vi "Main Tclk.vi"() -> ()   [LabVIEW 2018] (continued)
                n1472 = Multiply(x=w6714, y=w6704) -> (x*y=w6715:dbl)
                n1473 = local read "X full scale (V)"() -> (w6718:sgl)
                n1474 = Subtract(x=w6750, y="Y shift (nm/image)") -> (x-y=w6744:dbl)
                n1475 = expression code="x/1000"(w6744) -> (w6743:dbl)
                n1476 = Max & Min(x=0.1 ("upper limit"), y=w6715) -> (max(x,y)=w6708:dbl, min(x,y)=w6707:dbl)
                n1477 = Multiply(x=w6721, y=w6718) -> (x*y=w6722:dbl)
                n1478 = expression code="x/1000"("X shift (nm/image)") -> (w6745:sgl)
                n1479 = Select(t=w6722, s=w6720, f=w6717) -> (s? t:f=w6709:dbl)
                n1480 = Subtract(x=w6726, y=w6743) -> (x-y=w6753:dbl)
                n1481 = In Range and Coerce(upper limit=w6708, x=w6709, lower limit=w6707) -> (coerced(x)=w6705:dbl)  [unwired: 1 out]
                n1482 = Add(x=w6727, y=w6745) -> (x+y=w6748:sgl)
                n1483 = Multiply(x=w6703, y=w6704) -> (x*y=w6706:dbl)
                n1484 = Divide(x=w6706, y=w6705) -> (x/y=w6702:dbl)
                n1485 = Subtract(x=w6702, y=w6703) -> (x-y=w6742:dbl)
                n1486 = Subtract(x=w6702, y=w6710) -> (x-y=w6739:dbl)
                n1487 = expression code="x/2"(w6742) -> (w6741:dbl)
                n1488 = expression code="x/2"(w6739) -> (w6738:dbl)
                n1489 = Negate(x=w6741) -> (-x=w6740:dbl)
                n1490 = Negate(x=w6738) -> (-x=w6737:dbl)
                n1491 = In Range and Coerce(upper limit=w6741, x=w6748, lower limit=w6740) -> (coerced(x)=w6747:dbl)  [unwired: 1 out]
                n1492 = In Range and Coerce(upper limit=w6738, x=w6753, lower limit=w6737) -> (coerced(x)=w6752:dbl)  [unwired: 1 out]
                n1493 = local read "SEM Scan Parameters"() -> (w6757:T26)
                n1494 = Bundle By Name(cluster=w6757, "WD (mm)"=w6735, "X stig"=w6734, "Y stig"=w6733, "X aln"=w6732, "Y aln"=w6731, "X center (um)"=w6747, "Y center (um)"=w6752) -> (w6756:T26)
                n1495 = local write "SEM Scan Parameters"(w6756) -> ()
              }
              frame #17 {
                n1496 = local read "SEM Scan Parameters"() -> (w6879:T26)
                n1497 = local read "AF Count"() -> (w6875:u8)
                n1498 = local read "Auto Focus"() -> (w6881:bool)
                n1499 = Unbundle By Name(w6879) -> ("WD (mm)"=w6880:sgl[][])
                n1500 = case shown="True" w6881 {
                  tunnel: w6880 -> [w6889 w6899]
                  tunnel: [w6886 w6894] -> w6878
                  tunnel: [sgl[][][] [] ("Array") w6895] -> w6876
                  tunnel: w6875 -> [_ w6896]
                  frame False {
                    n1501 = local read "Milling para"() -> (w6891:T35)
                    n1502 = To Double Precision Float(number=w6889) -> (double precision float=w6885:dbl[][])
                    n1503 = Unbundle By Name(w6891) -> ("Z-step (nm)"=w6884:dbl, "Lines auto pause"=w6882:u16)
                    n1504 = expression code="1/sin(x/180*pi)"("FIB-SEM Angle") -> (w6890:dbl)
                    n1505 = expression code="x/1e6"(w6884) -> (w6883:dbl)
                    n1506 = Compound Arithmetic op=MULTIPLY(w6883, w6882, w6890) -> (w6893:dbl)
                    n1507 = Add(x=w6885, y=w6893) -> (x+y=w6888:dbl[][])
                    n1508 = To Single Precision Float(number=w6888) -> (single precision float=w6886:sgl[][])
                  }
                  frame True {
                    n1509 = property on="AF Steps" class="DigNum (strict)"("DisabledEnum"=T44."Disabled and Grayed Out" ("Disabled")) -> ()  [unwired: 2 in, 2 out]
                    n1510 = for {
                      tunnel: w6896 -> [w6905]
                      tunnel: w6899 -> [w6904] mode=indexing
                      tunnel: [w6903] -> w6898 mode=indexing
                      tunnel: [w6902] -> w6897 mode=indexing
                      i -> [w6901]
                      n1511 = for {
                        tunnel: w6905 -> [w6910]
                        tunnel: w6904 -> [w6913] mode=indexing
                        tunnel: [w6912] -> w6903 mode=indexing
                        tunnel: [w6911] -> w6902 mode=indexing
                        tunnel: w6901 -> [w6908]
                        i -> [w6906]
                        n1512 = Decrement(x=w6910) -> (x-1=w6907:u8)
                        n1513 = Equal To 0?(x=w6907) -> (x = 0?=w6909:bool)
                        n1514 = case shown="True" w6909 {
                          tunnel: [w6917 w6921] -> w6914
                          tunnel: w6913 -> [_ w6922]
                          tunnel: [w6917 w6921] -> w6911
                          tunnel: w6908 -> [w6916 _]
                          tunnel: w6906 -> [w6915 _]
                          frame False {
                            n1515 = local read "WD array tiled"() -> (w6918:sgl[][][])
                            n1516 = Index Array(array=w6918, index (dim 0)=w6916, index (dim 1)=w6915) -> (element=w6917:sgl[])  [unwired: 1 in]
                          }
                          frame True {
                            n1517 = local read "AF Range (nm)"() -> (w6920:sgl)
                            n1518 = local read "AF Steps"() -> (w6919:u8)
                            n1519 = expression code="x/1e6"(w6920) -> (w6923:sgl)
                            n1520 = call "Step down array.vi"("Steps"=w6919, "Range"=w6923, "Center"=w6922) -> ("Array"=w6921:dbl[])  [unwired: 8 in]
                          }
                        }
                        n1521 = Index Array(array=w6914, index=w6907) -> (element=w6912:dbl)
                      }
                    }
                    n1522 = To Single Precision Float(number=w6897) -> (single precision float=w6895:sgl[][][])
                    n1523 = To Single Precision Float(number=w6898) -> (single precision float=w6894:sgl[][])
                  }
                }
                n1524 = Bundle By Name(cluster=w6879, "WD (mm)"=w6878) -> (w6877:T26)
                n1525 = local write "WD array tiled"(w6876) -> ()
                n1526 = local write "SEM Scan Parameters"(w6877) -> ()
              }
              frame #18 {
                n1527 = local read "SEM Scan Parameters"() -> (w6931:T26)
                n1528 = local read "AS Count"() -> (w6925:u8)
                n1529 = local read "AA Count"() -> (w6924:u8)
                n1530 = Unbundle By Name(w6931) -> ("X stig"=w6934:sgl[][], "Y stig"=w6935:sgl[][])
                n1531 = Unbundle By Name(w6931) -> ("X aln"=w6937:sgl[][], "Y aln"=w6938:sgl[][])
                n1532 = case shown="\"Stig X\"" "Stig Options" {
                  tunnel: [w7005 w7012 w7038] -> w6930
                  tunnel: [w7004 w7009 w7040] -> w6929
                  tunnel: w6934 -> [w7005 w7010 w7038]
                  tunnel: w6935 -> [w7004 w7009 w7039]
                  tunnel: [w7003 w7008 dbl[][][] [] ("Array")] -> w6936
                  tunnel: [w7003 dbl[][][] [] ("Array") w7037] -> w6939
                  tunnel: w6925 -> [_ w7007 w7036]
                  frame "Defaut", Default {
                    w7003 = dbl[][][] [] ("Array")
                  }
                  frame "Stig X" {
                    n1533 = property on="AS Steps" class="DigNum (strict)"("DisabledEnum"=T44."Disabled and Grayed Out" ("Disabled")) -> ()  [unwired: 2 in, 2 out]
                    n1534 = for {
                      tunnel: w7007 -> [w7017]
                      tunnel: [w7016] -> w7012 mode=indexing
                      tunnel: w7010 -> [w7015] mode=indexing
                      tunnel: [w7014] -> w7008 mode=indexing
                      i -> [w7013]
                      n1535 = for {
                        tunnel: w7017 -> [w7022]
                        tunnel: [w7025] -> w7016 mode=indexing
                        tunnel: w7015 -> [w7024] mode=indexing
                        tunnel: [w7023] -> w7014 mode=indexing
                        tunnel: w7013 -> [w7019]
                        i -> [w7018]
                        n1536 = Decrement(x=w7022) -> (x-1=w7020:u8)
                        n1537 = Equal To 0?(x=w7020) -> (x = 0?=w7021:bool)
                        n1538 = case shown="False" w7021 {
                          tunnel: [w7027 w7033] -> w7026
                          tunnel: w7024 -> [_ w7034]
                          tunnel: [w7027 w7033] -> w7023
                          tunnel: w7019 -> [w7029 _]
                          tunnel: w7018 -> [w7028 _]
                          frame False {
                            n1539 = local read "StigX array tiled"() -> (w7030:sgl[][][])
                            n1540 = Index Array(array=w7030, index (dim 0)=w7029, index (dim 1)=w7028) -> (element=w7027:sgl[])  [unwired: 1 in]
                          }
                          frame True {
                            n1541 = local read "AS Range (%)"() -> (w7032:sgl)
                            n1542 = local read "AS Steps"() -> (w7031:u8)
                            n1543 = call "Step down array.vi"("Steps"=w7031, "Range"=w7032, "Center"=w7034) -> ("Array"=w7033:dbl[])  [unwired: 8 in]
                          }
                        }
                        n1544 = Index Array(array=w7026, index=w7020) -> (element=w7025:dbl)
                      }
                    }
                  }
                  frame "Stig Y" {
                    n1545 = property on="AS Steps" class="DigNum (strict)"("DisabledEnum"=T44."Disabled and Grayed Out" ("Disabled")) -> ()  [unwired: 2 in, 2 out]
                    n1546 = for {
                      tunnel: w7036 -> [w7046]
                      tunnel: [w7045] -> w7040 mode=indexing
                      tunnel: [w7044] -> w7037 mode=indexing
                      tunnel: w7039 -> [w7043] mode=indexing
                      i -> [w7042]
                      n1547 = for {
                        tunnel: w7046 -> [w7050]
                        tunnel: [w7054] -> w7045 mode=indexing
                        tunnel: [w7053] -> w7044 mode=indexing
                        tunnel: w7043 -> [w7052] mode=indexing
                        tunnel: w7042 -> [w7048]
                        i -> [w7047]
                        n1548 = Decrement(x=w7050) -> (x-1=w7049:u8)
                        n1549 = Equal To 0?(x=w7049) -> (x = 0?=w7051:bool)
                        n1550 = case shown="False" w7051 {
                          tunnel: [w7056 w7061] -> w7055
                          tunnel: [w7056 w7061] -> w7053
                          tunnel: w7052 -> [_ w7060]
                          tunnel: w7048 -> [w7058 _]
                          tunnel: w7047 -> [w7057 _]
                          frame False {
                            n1551 = local read "StigY array tiled"() -> (w7059:sgl[][][])
                            n1552 = Index Array(array=w7059, index (dim 0)=w7058, index (dim 1)=w7057) -> (element=w7056:sgl[])  [unwired: 1 in]
                          }
                          frame True {
                            n1553 = local read "AS Range (%)"() -> (w7062:sgl)
                            n1554 = local read "AS Steps"() -> (w7063:u8)
                            n1555 = call "Step down array.vi"("Steps"=w7063, "Range"=w7062, "Center"=w7060) -> ("Array"=w7061:dbl[])  [unwired: 8 in]
                          }
                        }
                        n1556 = Index Array(array=w7055, index=w7049) -> (element=w7054:dbl)
                      }
                    }
                  }
                }
                n1557 = case shown="\"Aln Y\"" "Aln Options" {
                  tunnel: [w6944 w6951 w6979] -> w6928
                  tunnel: [w6943 w6947 w6977] -> w6927
                  tunnel: w6937 -> [w6944 w6949 w6979]
                  tunnel: w6938 -> [w6943 w6947 w6978]
                  tunnel: [w6942 w6948 dbl[][][] [] ("Array")] -> w6940
                  tunnel: [w6942 dbl[][][] [] ("Array") w6976] -> w6941
                  tunnel: w6924 -> [_ w6946 w6975]
                  frame "Defaut", Default {
                    w6942 = dbl[][][] [] ("Array")
                  }
                  frame "Aln X" {
                    n1558 = property on="AA Steps" class="DigNum (strict)"("DisabledEnum"=T44."Disabled and Grayed Out" ("Disabled")) -> ()  [unwired: 2 in, 2 out]
                    n1559 = for {
                      tunnel: [w6956] -> w6951 mode=indexing
                      tunnel: w6949 -> [w6955] mode=indexing
                      tunnel: [w6954] -> w6948 mode=indexing
                      tunnel: w6946 -> [w6953]
                      i -> [w6952]
                      n1560 = for {
                        tunnel: [w6964] -> w6956 mode=indexing
                        tunnel: w6955 -> [w6963] mode=indexing
                        tunnel: [w6962] -> w6954 mode=indexing
                        tunnel: w6953 -> [w6961]
                        tunnel: w6952 -> [w6958]
                        i -> [w6957]
                        n1561 = Decrement(x=w6961) -> (x-1=w6959:u8)
                        n1562 = Equal To 0?(x=w6959) -> (x = 0?=w6960:bool)
                        n1563 = case shown="False" w6960 {
                          tunnel: [w6966 w6972] -> w6965
                          tunnel: w6963 -> [_ w6973]
                          tunnel: [w6966 w6972] -> w6962
                          tunnel: w6958 -> [w6967 _]
                          tunnel: w6957 -> [w6968 _]
                          frame False {
                            n1564 = local read "AlnX array tiled"() -> (w6969:sgl[][][])
                            n1565 = Index Array(array=w6969, index (dim 0)=w6967, index (dim 1)=w6968) -> (element=w6966:sgl[])  [unwired: 1 in]
                          }
                          frame True {
                            n1566 = local read "AA Range (%)"() -> (w6970:sgl)
                            n1567 = local read "AA Steps"() -> (w6971:u8)
                            n1568 = call "Step down array.vi"("Steps"=w6971, "Range"=w6970, "Center"=w6973) -> ("Array"=w6972:dbl[])  [unwired: 8 in]
                          }
                        }
                        n1569 = Index Array(array=w6965, index=w6959) -> (element=w6964:dbl)
                      }
                    }
                  }
                  frame "Aln Y" {
                    n1570 = property on="AA Steps" class="DigNum (strict)"("DisabledEnum"=T44."Disabled and Grayed Out" ("Disabled")) -> ()  [unwired: 2 in, 2 out]
                    n1571 = for {
                      tunnel: w6975 -> [w6985]
                      tunnel: w6978 -> [w6984] mode=indexing
                      tunnel: [w6983] -> w6977 mode=indexing
                      tunnel: [w6982] -> w6976 mode=indexing
                      i -> [w6981]
                      n1572 = for {
                        tunnel: w6985 -> [w6990]
                        tunnel: w6984 -> [w6993] mode=indexing
                        tunnel: [w6992] -> w6983 mode=indexing
                        tunnel: [w6991] -> w6982 mode=indexing
                        tunnel: w6981 -> [w6987]
                        i -> [w6986]
                        n1573 = Decrement(x=w6990) -> (x-1=w6989:u8)
                        n1574 = Equal To 0?(x=w6989) -> (x = 0?=w6988:bool)
                        n1575 = case shown="False" w6988 {
                          tunnel: [w6995 w6999] -> w6994
                          tunnel: w6993 -> [_ w7000]
                          tunnel: [w6995 w6999] -> w6991
                          tunnel: w6987 -> [w6996 _]
                          tunnel: w6986 -> [w6997 _]
                          frame False {
                            n1576 = local read "AlnY array tiled"() -> (w6998:sgl[][][])
                            n1577 = Index Array(array=w6998, index (dim 0)=w6996, index (dim 1)=w6997) -> (element=w6995:sgl[])  [unwired: 1 in]
                          }
                          frame True {
                            n1578 = local read "AA Steps"() -> (w7002:u8)
                            n1579 = local read "AA Range (%)"() -> (w7001:sgl)
                            n1580 = call "Step down array.vi"("Steps"=w7002, "Range"=w7001, "Center"=w7000) -> ("Array"=w6999:dbl[])  [unwired: 8 in]
                          }
                        }
                        n1581 = Index Array(array=w6994, index=w6989) -> (element=w6992:dbl)
                      }
                    }
                  }
                }
                n1582 = local write "StigX array tiled"(w6936) -> ()
                n1583 = local write "StigY array tiled"(w6939) -> ()
                n1584 = local write "AlnX array tiled"(w6940) -> ()
                n1585 = local write "AlnY array tiled"(w6941) -> ()
                n1586 = Bundle By Name(cluster=w6931, "X stig"=w6930, "Y stig"=w6929, "X aln"=w6928, "Y aln"=w6927) -> (w6926:T26)
                n1587 = local write "SEM Scan Parameters"(w6926) -> ()
              }
              frame #19 {
                n1588 = local read "Tiled scan inputs"() -> (w7073:T6)
                n1589 = local read "SEM HW Config"() -> (w7074:T9)
                n1590 = local read "Detector Information"() -> (w7075:T8)
                n1591 = local read "SEM Scan Parameters"() -> (w7076:T26)
                n1592 = local read "SEM Options"() -> (w7077:T27)
                n1593 = local read "Focus Index Options"() -> (w7071:T28)
                n1594 = local read "File Information"() -> (w7078:T31)
                n1595 = local read "SEM-FIB Delay (s)"() -> (w7066:u32)
                n1596 = local read "After SEM"() -> (w7069:bool)
                n1597 = local read "FIB"() -> (w7068:bool)
                n1598 = local read "Milling para"() -> (w7079:T35)
                n1599 = local read "Additional Info"() -> (w7064:cluster{"Restart flag":u8, "Stage move flag":u8})
                n1600 = Not(x=w7069) -> (.not. x?=w7065:bool)
                n1601 = Greater Than 0?(x=w7066) -> (x > 0?=w7067:bool)
                n1602 = Compound Arithmetic op=AND(w7067, w7065, w7068) -> (w7070:bool)
                n1603 = Bundle By Name(cluster=w7073, "HW Config"=w7074, "Det Info"=w7075, "SEM Scan Parameters"=w7076, "SEM Options"=w7077, "Focus Index Options"=w7071, "File Information"=w7078, "Milling para"=w7079, "Additional Info"=w7064) -> (w7072:T6)
                n1604 = case shown="True" w7070 {
                  tunnel: w7066 -> [_ w7080]
                  frame False {
                  }
                  frame True {
                    n1605 = local read "FIB blank condenser %"() -> (w7089:u8)
                    n1606 = expression code="x*10"(w7080) -> (w7081:u32)
                    n1607 = Number To Decimal String(number=w7080) -> (decimal integer string=w7082:string)  [unwired: 1 in]
                    n1608 = for {
                      N: w7081 -> [_]
                      stop <- w7092 stop-if-true
                      n1609 = local read "Mill Manual Pause"() -> (w7093:bool)
                      n1610 = local read "FIB"() -> (w7095:bool)
                      n1611 = Wait Until Next ms Multiple(millisecond multiple=u32 100) -> ()  [unwired: 1 out]
                      n1612 = Not(x=w7095) -> (.not. x?=w7094:bool)
                      n1613 = Or(x=w7094, y=w7093) -> (x .or. y?=w7092:bool)
                    }
                    n1614 = Less?(x=w7089, y=u8 100) -> (x < y?=w7091:bool)
                    n1615 = Greater Or Equal?(x=w7080, y=5.0) -> (x >= y?=w7090:bool)
                    n1616 = To Single Precision Float(number=w7089) -> (single precision float=w7088:sgl)
                    n1617 = Compound Arithmetic op=AND(w7091, w7090) -> (w7087:bool)
                    n1618 = Concatenate Strings(w7082, " s delay after FIB milling..." ("string")) -> (w7084:string)
                    n1619 = local write "Status message"(w7084) -> ()
                    n1620 = case shown="True" w7087 {
                      tunnel: w7088 -> [_ w7098]
                      tunnel: w7080 -> [_ w7097]
                      frame False {
                      }
                      frame True {
                        n1621 = stacked-sequence {
                          seq-local: [w7100 _ _ _] -> [_ w7108 _ _]
                          seq-local: [w7099 _ _ _] -> [_ w7106 _ w7117]
                          seq-local: [_ w7107 _ _] -> [_ _ _ w7118]
                          tunnel: w7098 -> [_ w7105 _ _]
                          tunnel: w7097 -> [_ _ w7111 _]
                          frame #0 {
                            n1622 = local read "Api"() -> (w7102:refnum<k7>)
                            n1623 = call "SmartSEM Remote API get float.vi"("lpszParam"="AP_FIB_CONDENSER" ("Status message"), "ActiveX Container"=w7102) -> ("vValue"=w7099:sgl, "reference out"=w7100:refnum<k7>)  [unwired: 7 in, 1 out]
                          }
                          frame #1 {
                            n1624 = Compound Arithmetic op=MULTIPLY(w7106, w7105, sgl 0.01 ("value")) -> (w7104:sgl)
                            n1625 = call "SmartSEM Remote API set float.vi"("vValue"=w7104, "lpszParam"="AP_FIB_CONDENSER" ("Status message"), "ActiveX Container"=w7108) -> ("reference out"=w7107:refnum<k7>)  [unwired: 7 in, 1 out]
                          }
                          frame #2 {
                            n1626 = expression code="(x-3)*10"(w7111) -> (w7110:u32)
                            n1627 = for {
                              N: w7110 -> [_]
                              stop <- w7112 stop-if-true
                              n1628 = local read "Mill Manual Pause"() -> (w7113:bool)
                              n1629 = local read "FIB"() -> (w7115:bool)
                              n1630 = Wait Until Next ms Multiple(millisecond multiple=u32 100) -> ()  [unwired: 1 out]
                              n1631 = Not(x=w7115) -> (.not. x?=w7114:bool)
                              n1632 = Or(x=w7114, y=w7113) -> (x .or. y?=w7112:bool)
                            }
                          }
                          frame #3 {
                            n1633 = call "SmartSEM Remote API set float.vi"("vValue"=w7117, "lpszParam"="AP_FIB_CONDENSER" ("Status message"), "ActiveX Container"=w7118) -> ()  [unwired: 7 in, 2 out]
                          }
                        }
                      }
                    }
                  }
                }
                n1634 = local write "Tiled scan inputs"(w7072) -> ()
              }
              frame #20 {
                n1635 = local read "Mill Stop"() -> (w7121:bool)
                n1636 = local read "FIB"() -> (w7124:bool)
                n1637 = local read "Stop"() -> (w7125:bool)
                n1638 = Not(x=w7125) -> (.not. x?=w7123:bool)
                n1639 = Not(x=w7121) -> (.not. x?=w7120:bool)
                n1640 = Compound Arithmetic op=AND(w7120, w7124, w7123) -> (w7122:bool)
                n1641 = case shown="True" w7122 {
                  frame False {
                  }
                  frame True {
                    w7182 = TRUE ("SEM Options.Set WD")
                    n1642 = local read "WatchDog Mode"() -> (w7144:u16)
                    n1643 = local read "Api"() -> (w7138:refnum<k7>)
                    n1644 = local read "Tiled scan inputs"() -> (w7186:T6)
                    n1645 = Bundle By Name(cluster=w7186, "SEM Options.Set WD"=w7182, "SEM Options.Set stig"=w7182, "SEM Options.Set aln"=w7182, "SEM Options.Freeze"=w7182) -> (w7139:T6)
                    n1646 = call "2D scan tiled.vi"("WatchDog Mode"=w7144, "Tiled scan inputs"=w7139, "ActiveX Container"=w7138) -> ("Image Focus Index Tiled"=w7181:T53, "Image Focus Index Array Tiled"=w7180:T54, "Low res scale Tiled (um/pix)"=→"Low res scale tiled":dbl[][], "Single scan outputs"=w7185:T55, "SEM Spec. I Tiled (nA)"=w7160:sgl[][], "8-bit over scale"=w7170:bool[])  [unwired: 3 in]
                    n1647 = Array Size(array=w7160) -> (size(s)=w7161:i32[])
                    n1648 = Multiply Array Elements(1:w7161) -> (0:w7162:i32)
                    n1649 = local read "FI Detector"() -> (w7194:u16)
                    n1650 = Reshape Array(w7160, w7162) -> (w7163:sgl[])
                    n1651 = call-poly <vilib>:"Mean.vi"("X"=w7163) -> ("mean"=→"SEM Specimen I":dbl)  [unwired: 1 out]
                    n1652 = Unbundle By Name(w7185) -> ("SEM Parameters"=w7184:T13, "Image Focus Index"=w7176:T14, "FIB parameters"=→"FIB Parameters":T56)
                    n1653 = case shown="0, Default" w7194 {
                      tunnel: w7181 -> [w7255 w7259 w7263 w7267]
                      tunnel: [w7254 w7256 w7262 w7266] -> w7204
                      tunnel: w7180 -> [w7253 w7258 w7261 w7265]
                      tunnel: [w7252 w7257 w7260 w7264] -> w7203
                      frame 0, Default {
                        n1654 = Unbundle By Name(w7255) -> ("A Img Focus Index"=w7254:sgl[][])
                        n1655 = Unbundle By Name(w7253) -> ("A Img Focus Index array"=w7252:sgl[][][][])
                      }
                      frame 1 {
                        n1656 = Unbundle By Name(w7259) -> ("B Img Focus Index"=w7256:sgl[][])
                        n1657 = Unbundle By Name(w7258) -> ("B Img Focus Index array"=w7257:sgl[][][][])
                      }
                      frame 2 {
                        n1658 = Unbundle By Name(w7263) -> ("C Img Focus Index"=w7262:sgl[][])
                        n1659 = Unbundle By Name(w7261) -> ("C Img Focus Index array"=w7260:sgl[][][][])
                      }
                      frame 3 {
                        n1660 = Unbundle By Name(w7267) -> ("D Img Focus Index"=w7266:sgl[][])
                        n1661 = Unbundle By Name(w7265) -> ("D Img Focus Index array"=w7264:sgl[][][][])
                      }
                    }
                    "Focus Index tiled" <- w7204
                    "Focus Index array tiled" <- w7203
                    n1662 = local read "Pause for reheat"() -> (w7137:bool)
                    n1663 = local write "SEM Parameters"(w7184) -> ()
                    n1664 = local write "Image Focus Index"(w7176) -> ()
                    n1665 = Index Array(array=w7170, index #1=0 ("index"), index #2=1 ("index")) -> (element #1=w7173:bool, element #2=w7174:bool)
                    n1666 = Select(t="Pausing for FIB reheat ..." ("Status message"), s=w7137, f="SEM between FIB" ("Status message")) -> (s? t:f=w7146:string)
                    n1667 = local write "Det A over scale"(w7173) -> ()
                    n1668 = local write "Det B over scale"(w7174) -> ()
                    n1669 = Array Size(array=w7204) -> (size(s)=w7179:i32[])
                    n1670 = Not(x=w7137) -> (.not. x?=w7133:bool)
                    n1671 = local write "Status message"(w7146) -> ()
                    n1672 = local read "SEM scan time"() -> (w7131:dbl)
                    n1673 = Multiply Array Elements(1:w7179) -> (0:w7178:i32)
                    n1674 = Reshape Array(w7204, w7178) -> (w7177:sgl[])
                    n1675 = call-poly <vilib>:"Mean.vi"("X"=w7177) -> ("mean"=→"Focus Index":dbl)  [unwired: 1 out]
                    n1676 = Greater Or Equal?(x=w7131, y=6.0) -> (x >= y?=w7135:bool)
                    n1677 = Less?(x="FIB blank condenser %", y=u8 100) -> (x < y?=w7130:bool)
                    n1678 = To Single Precision Float(number="FIB blank condenser %") -> (single precision float=w7127:sgl)
                    n1679 = Compound Arithmetic op=AND(w7130, w7133, w7135) -> (w7134:bool)
                    n1680 = case shown="True" w7134 {
                      tunnel: w7131 -> [w7205 w7220]
                      tunnel: [w7206 w7219] -> w7132
                      tunnel: w7127 -> [_ w7218]
                      frame False {
                        w7210 = 10.0 ("rate")
                        n1681 = In Range and Coerce(upper limit=60.0, x=w7205, lower limit=2.0) -> (coerced(x)=w7211:dbl)  [unwired: 1 out]
                        n1682 = Multiply(x=w7211, y=w7210) -> (x*y=w7212:dbl)
                        n1683 = for {
                          N: w7212 -> [_]
                          shift-right: [w7217] -> w7206
                          shift-left: sgl[][] [] -> [w7216]
                          tunnel: w7210 -> [w7214]
                          n1684 = shared-variable ".\\Zeiss Library.lvlib\\Logs"() -> (w7213:sgl[])  [unwired: 1 in, 1 out]
                          n1685 = expression code="1000/x"(w7214) -> (w7215:dbl)
                          n1686 = Wait Until Next ms Multiple(millisecond multiple=w7215) -> ()  [unwired: 1 out]
                          n1687 = Build Array (concatenate)(w7216, w7213) -> (w7217:sgl[][])
                        }
                      }
                      frame True {
                        n1688 = stacked-sequence {
                          seq-local: [w7222 _ _ _ _ _] -> [_ w7230 _ _ _ _]
                          seq-local: [w7221 _ _ _ _ _] -> [_ w7228 _ w7234 _ _]
                          seq-local: [_ w7229 _ _ _ _] -> [_ _ _ w7235 _ _]
                          tunnel: w7220 -> [_ _ w7233 _ _ _]
                          tunnel: [_ _ _ _ _ w7239] -> w7219
                          tunnel: w7218 -> [_ w7227 _ _ _ _]
                          frame #0 {
                            n1689 = local read "Api"() -> (w7224:refnum<k7>)
                            n1690 = call "SmartSEM Remote API get float.vi"("lpszParam"="AP_FIB_CONDENSER" ("Status message"), "ActiveX Container"=w7224) -> ("vValue"=w7221:sgl, "reference out"=w7222:refnum<k7>)  [unwired: 7 in, 1 out]
                          }
                          frame #1 {
                            n1691 = Compound Arithmetic op=MULTIPLY(w7228, w7227, sgl 0.01 ("value")) -> (w7226:sgl)
                            n1692 = call "SmartSEM Remote API set float.vi"("vValue"=w7226, "lpszParam"="AP_FIB_CONDENSER" ("Status message"), "ActiveX Container"=w7230) -> ("reference out"=w7229:refnum<k7>)  [unwired: 7 in, 1 out]
                          }
                          frame #2 {
                            n1693 = expression code="(x-4)*1000"(w7233) -> (w7232:dbl)
                            n1694 = Wait (ms)(milliseconds to wait=w7232) -> ()  [unwired: 1 out]
                          }
                          frame #3 {
                            n1695 = call "SmartSEM Remote API set float.vi"("vValue"=w7234, "lpszParam"="AP_FIB_CONDENSER" ("Status message"), "ActiveX Container"=w7235) -> ()  [unwired: 7 in, 2 out]
                          }
                          frame #4 {
                            n1696 = Wait (ms)(milliseconds to wait=u32 1000) -> ()  [unwired: 1 out]
                          }
                          frame #5 {
                            n1697 = for {
                              N: 20 -> [_]
                              shift-right: [w7244] -> w7239
                              shift-left: sgl[][] [] -> [w7243]
                              n1698 = shared-variable ".\\Zeiss Library.lvlib\\Logs"() -> (w7242:sgl[])  [unwired: 1 in, 1 out]
                              n1699 = Wait Until Next ms Multiple(millisecond multiple=u32 100) -> ()  [unwired: 1 out]
                              n1700 = Build Array (concatenate)(w7243, w7242) -> (w7244:sgl[][])
                            }
                          }
                        }
                      }
                    }
                    n1701 = shared-variable ".\\Zeiss Library.lvlib\\Faraday cup offset"() -> (w7165:sgl)  [unwired: 1 in, 1 out]
                    n1702 = local read "Alert Settings"() -> (w7158:T36)
                    n1703 = Unbundle By Name(w7158) -> ("Low limit (F)"=w7152:sgl, "High limit (F)"=w7153:sgl)
                    n1704 = local read "Machine Type"() -> (w7191:u8)
                    n1705 = local read "Faraday Cup array"() -> (w7202:sgl[])
                    n1706 = local read "Specimen I array"() -> (w7201:sgl[])
                    n1707 = shared-variable ".\\Zeiss Library.lvlib\\Specimen (nA)"() -> (w7143:sgl)  [unwired: 1 in, 1 out]
                    "Specimen I (nA)" <- w7143
                    n1708 = shared-variable ".\\Zeiss Library.lvlib\\Beam Dump 1 (nA)"() -> (w7142:sgl)  [unwired: 1 in, 1 out]
                    "Beam Dump 1 (nA)" <- w7142
                    n1709 = shared-variable ".\\Zeiss Library.lvlib\\Beam Dump 2 (nA)"() -> (w7141:sgl)  [unwired: 1 in, 1 out]
                    "Beam Dump 2 (nA)" <- w7141
                    n1710 = local read "Milling I array"() -> (w7167:sgl[])
                    n1711 = shared-variable ".\\Zeiss Library.lvlib\\Milling I (nA)"() -> (w7140:sgl)  [unwired: 1 in, 1 out]
                    "Milling I (nA)" <- w7140
                    n1712 = local read "Temp low limit array"() -> (w7156:sgl[])
                    n1713 = local read "Temp high limit array"() -> (w7155:sgl[])
                    n1714 = local read "Beam Dump 1 array"() -> (w7200:sgl[])
                    n1715 = local read "Beam Dump 2 array"() -> (w7168:sgl[])
                    n1716 = local read "Temp array"() -> (w7199:sgl[])
                    n1717 = local read "Temp (F)"() -> (w7187:sgl)
                    n1718 = shared-variable ".\\Zeiss Library.lvlib\\Temp (F)"(w7187) -> ()  [unwired: 1 in, 1 out]
                    n1719 = Build Array (concatenate)(w7201, w7143) -> (w7197:sgl[])
                    n1720 = Build Array (concatenate)(w7199, w7187) -> (w7192:sgl[])
                    n1721 = Build Array (concatenate)(w7200, w7142) -> (w7196:sgl[])
                    n1722 = Build Array (concatenate)(w7168, w7141) -> (w7169:sgl[])
                    n1723 = Build Array (concatenate)(w7167, w7140) -> (w7166:sgl[])
                    n1724 = Build Array (concatenate)(w7156, w7152) -> (w7157:sgl[])
                    n1725 = Build Array (concatenate)(w7155, w7153) -> (w7154:sgl[])
                    n1726 = Delete From Array(array=w7132, length=15.0 ("rate"), index (row)=0 ("disabled index (col)")) -> (array with subset deleted=w7151:sgl[][])  [unwired: 1 in, 1 out]
                    n1727 = local write "Temp array"(w7192) -> ()
                    n1728 = local write "Specimen I array"(w7197) -> ()
                    n1729 = local write "Milling I array"(w7166) -> ()
                    n1730 = local write "Temp low limit array"(w7157) -> ()
                    n1731 = local write "Temp high limit array"(w7154) -> ()
                    n1732 = local write "Beam Dump 1 array"(w7196) -> ()
                    n1733 = local write "Beam Dump 2 array"(w7169) -> ()
                    n1734 = Transpose 2D Array(2D array=w7151) -> (transposed array=w7193:sgl[][])
                    n1735 = for {
                      tunnel: [w7251] -> w7189 mode=indexing
                      tunnel: w7193 -> [w7250] mode=indexing
                      n1736 = call-poly <vilib>:"Basic Averaged DC-RMS.vi"("signal in"=w7250) -> ("DC value"=w7251:dbl)  [unwired: 7 in, 3 out]
                    }
                    n1737 = To Single Precision Float(number=w7189) -> (single precision float=w7195:sgl[])
                    n1738 = Index Array(array=w7195) -> (element=w7149:sgl)  [unwired: 1 in]
                    n1739 = Subtract(x=w7149, y=w7165) -> (x-y=w7190:sgl)
                    n1740 = case shown="2" w7191 {
                      tunnel: w7190 -> [w7245 _ _]
                      tunnel: [w7245 w7248 w7249] -> w7188
                      tunnel: w7142 -> [_ w7247 _]
                      tunnel: w7143 -> [_ w7246 _]
                      tunnel: w7149 -> [_ _ w7249]
                      frame 0, Default {
                      }
                      frame 1 {
                        n1741 = Subtract(x=w7247, y=w7246) -> (x-y=w7248:sgl)
                      }
                      frame 2 {
                      }
                    }
                    "Faraday Cup (nA)" <- w7188
                    n1742 = shared-variable ".\\Zeiss Library.lvlib\\Faraday Cup (nA)"(w7188) -> ()  [unwired: 1 in, 1 out]
                    n1743 = Build Array (concatenate)(w7202, w7188) -> (w7198:sgl[])
                    n1744 = local write "Faraday Cup array"(w7198) -> ()
                    "FRC resolution" <- sgl 0.0 ("FRC resolution")
                  }
                }
              }
              frame #21 {
                n1745 = local read "FI array for stop limit"() -> (w7309:sgl[])
                n1746 = local read "Focus Index"() -> (w7279:sgl)
                n1747 = local read "Milling para"() -> (w7276:T35)
                n1748 = local read "Machine Type"() -> (w7275:u8)
                n1749 = local read "Alert Settings"() -> (w7300:T36)
                n1750 = Unbundle By Name(w7276) -> ("FIB PID measured"=w7277:u8, "FIB PID target"=w7268:sgl)
                n1751 = Unbundle By Name(w7300) -> ("FI stop limit auto"=w7303:bool)
                n1752 = local read "Auto re-engage"() -> (w7272:bool)
                n1753 = Build Array (concatenate)(w7309, w7279) -> (w7301:sgl[])
                n1754 = Unbundle By Name(w7300) -> ("FI low limit auto"=w7307:bool)
                n1755 = local write "FI array for stop limit"(w7301) -> ()
                n1756 = Array Size(array=w7301) -> (size(s)=w7306:i32)
                n1757 = case shown="2" w7277 {
                  tunnel: w7275 -> [w7342 _ w7346 _]
                  tunnel: [w7341 0.5 ("Minimum half range") w7347 0.5 ("Minimum half range")] -> w7274
                  frame 0 {
                    n1758 = case shown="2" w7342 {
                      tunnel: [0.5 ("Minimum half range") 0.8 ("Minimum half range")] -> w7341
                      frame 0, Default {
                      }
                      frame 2 {
                      }
                    }
                  }
                  frame 1 {
                  }
                  frame 2 {
                    n1759 = case shown="2" w7346 {
                      tunnel: [0.3 ("Minimum half range") 0.6 ("Minimum half range")] -> w7347
                      frame 0, Default {
                      }
                      frame 2 {
                      }
                    }
                  }
                  frame 3, Default {
                  }
                }
                n1760 = Or(x=w7303, y=w7272) -> (x .or. y?=w7302:bool)
                n1761 = Greater Or Equal?(x=w7306, y=5 ("x")) -> (x >= y?=w7304:bool)
                n1762 = And(x=w7304, y=w7302) -> (x .and. y?=w7271:bool)
                n1763 = And(x=w7304, y=w7307) -> (x .and. y?=w7308:bool)
                n1764 = local read "Focus index array"() -> (w7286:sgl[])
                n1765 = case shown="True" w7308 {
                  tunnel: w7300 -> [w7351 w7361]
                  tunnel: w7301 -> [_ w7358]
                  tunnel: [w7351 w7352] -> w7270
                  frame False {
                  }
                  frame True {
                    w7357 = 0.2 ("Minimum half range")
                    n1766 = call "Auto limits.vi"("lower band factor"=w7357, "upper band factor"=w7357, "Method"="sqrt of mean", "Minimum half range"=0.1, "Length"=5, "Input array"=w7358) -> ("Low limit"=w7356:dbl)  [unwired: 3 in, 2 out]
                    n1767 = Max & Min(x=w7356, y=0.0) -> (max(x,y)=w7353:dbl)  [unwired: 1 out]
                    n1768 = Bundle By Name(cluster=w7361, "Focus index low limit"=w7353) -> (w7352:T36)
                    n1769 = local write "Alert Settings"(w7352) -> ()
                  }
                }
                n1770 = case shown="True" w7271 {
                  tunnel: w7270 -> [_ w7312]
                  tunnel: w7301 -> [_ w7319]
                  frame False {
                  }
                  frame True {
                    w7314 = 0.4 ("Minimum half range")
                    n1771 = call "Auto limits.vi"("lower band factor"=w7314, "upper band factor"=w7314, "Method"="sqrt of mean", "Minimum half range"=0.4, "Length"=10, "Input array"=w7319) -> ("Low limit"=w7318:dbl)  [unwired: 3 in, 2 out]
                    n1772 = Unbundle By Name(w7312) -> ("Focus index low limit"=w7311:sgl)
                    n1773 = Max & Min(x=w7318, y=0.0) -> ()  [unwired: 2 out]
                    n1774 = expression code="x*0.75"(w7311) -> (w7310:sgl)
                    n1775 = Bundle By Name(cluster=w7312, "Focus index stop limit"=w7310) -> (w7320:T36)
                    n1776 = local write "Alert Settings"(w7320) -> ()
                  }
                }
                n1777 = case shown="True" w7272 {
                  tunnel: [w7322 w7328] -> w7273
                  tunnel: w7274 -> [w7322 w7329]
                  tunnel: [1.0 ("Minimum half range") w7327] -> w7269
                  tunnel: w7268 -> [_ w7326]
                  frame False {
                  }
                  frame True {
                    n1778 = local read "Re-engage counts"() -> (w7330:u8)
                    n1779 = expression code="x*0.15"(w7326) -> (w7325:sgl)
                    n1780 = Max & Min(x=sgl 1.0, y=w7325) -> (max(x,y)=w7323:sgl)  [unwired: 1 out]
                    n1781 = case shown="1" w7330 {
                      tunnel: [w7332 w7336 w7340] -> w7328
                      tunnel: w7329 -> [w7332 w7335 w7339]
                      tunnel: [1.0 ("Minimum half range") w7334 w7338] -> w7327
                      tunnel: w7323 -> [_ w7333 w7337]
                      frame 0, Default {
                      }
                      frame 1 {
                        w7334 = 4.0 ("Minimum half range")
                        n1782 = Compound Arithmetic op=MULTIPLY(w7335, w7333, w7334) -> (w7336:dbl)
                      }
                      frame 2 {
                        w7338 = 2.0 ("Minimum half range")
                        n1783 = Compound Arithmetic op=MULTIPLY(w7339, w7337, w7338) -> (w7340:dbl)
                      }
                    }
                  }
                }
                "FIB CL control band" <- w7273
                "FIB CL control band factor" <- w7269
                n1784 = Build Array (concatenate)(w7286, w7279) -> (w7280:sgl[])
                n1785 = local write "Focus index array"(w7280) -> ()
                n1786 = Unbundle By Name(w7270) -> ("Focus index low limit"=w7278:sgl)
                n1787 = local read "Auto Focus"() -> (w7297:bool)
                n1788 = local read "Auto Stig"() -> (w7298:bool)
                n1789 = local read "Auto Align"() -> (w7293:bool)
                n1790 = Divide(x="Smart upload FI threshold", y=100.0) -> (x/y=w7283:dbl)
                n1791 = Not(x=w7297) -> (.not. x?=w7292:bool)
                n1792 = Not(x=w7298) -> (.not. x?=w7291:bool)
                n1793 = Not(x=w7293) -> (.not. x?=w7290:bool)
                n1794 = Less Or Equal?(x=w7279, y=w7278) -> (x <= y?=w7294:bool)
                n1795 = Compound Arithmetic op=AND(w7292, w7291, w7290) -> (w7289:bool)
                n1796 = Multiply(x=w7278, y=w7283) -> (x*y=w7281:dbl)
                n1797 = Compound Arithmetic op=AND(w7294, w7289) -> (→"Focus index warning active":bool)
                n1798 = Greater Or Equal?(x=w7281, y=w7279) -> (x >= y?=→"Smart upload fail":bool)
                n1799 = local read "FI low limit array"() -> (w7287:sgl[])
                n1800 = Greater?(x=w7279, y=w7278) -> (0:w7296:bool)
                n1801 = Build Array (concatenate)(w7287, w7278) -> (w7288:sgl[])
                n1802 = Compound Arithmetic op=AND(w7296, w7289) -> (→"Focus index recovery active":bool)
                n1803 = local write "FI low limit array"(w7288) -> ()
              }
              frame #22 {
                n1804 = local read "Auto Align"() -> (w7368:bool)
                n1805 = local read "Auto Focus"() -> (w7364:bool)
                n1806 = local read "Auto Stig"() -> (w7367:bool)
                n1807 = local read "Focus Index tiled"() -> (w7365:sgl[][])
                n1808 = local read "Focus Index array tiled"() -> (w7366:sgl[][][][])
                n1809 = for {
                  tunnel: w7365 -> [w7376] mode=indexing
                  tunnel: [w7375] -> w7363 mode=indexing
                  tunnel: [w7374] -> w7362 mode=indexing
                  tunnel: w7364 -> [w7373]
                  tunnel: w7366 -> [w7372] mode=indexing
                  tunnel: w7367 -> [w7371]
                  tunnel: w7368 -> [w7370]
                  i -> [w7369]
                  n1810 = for {
                    tunnel: w7376 -> [w7386] mode=indexing
                    tunnel: [w7385] -> w7375 mode=indexing
                    tunnel: [w7384] -> w7374 mode=indexing
                    tunnel: w7373 -> [w7381]
                    tunnel: w7372 -> [w7383] mode=indexing
                    tunnel: w7371 -> [w7380]
                    tunnel: w7370 -> [w7379]
                    tunnel: w7369 -> [w7378]
                    i -> [w7377]
                    n1811 = Compound Arithmetic op=OR(w7381, w7380, w7379) -> (w7382:bool)
                    n1812 = case shown="False" w7382 {
                      tunnel: w7386 -> [_ w7412]
                      tunnel: w7383 -> [_ w7411]
                      tunnel: [w7388 w7410] -> w7385
                      tunnel: [w7387 w7409] -> w7384
                      tunnel: w7381 -> [_ w7406]
                      tunnel: w7380 -> [_ w7404]
                      tunnel: w7379 -> [_ w7402]
                      tunnel: w7378 -> [_ w7394]
                      tunnel: w7377 -> [_ w7393]
                      frame False {
                        n1813 = local read "FI grid array"() -> (w7387:sgl[][][])
                        n1814 = local read "FI array"() -> (w7388:sgl[])
                      }
                      frame True {
                        w7408 = u8 1 ("AF Count")
                        n1815 = local read "AF Count"() -> (w7391:u8)
                        n1816 = local read "AS Count"() -> (w7389:u8)
                        n1817 = local read "AA Count"() -> (w7390:u8)
                        n1818 = local read "FI array tiled"() -> (w7397:sgl[][][])
                        n1819 = local read "FI grid array tiled"() -> (w7395:sgl[][][][][])
                        n1820 = Index Array(array=w7397, index (dim 0)=w7394, index (dim 1)=w7393) -> (element=w7396:sgl[])  [unwired: 1 in]
                        n1821 = Index Array(array=w7395, index (dim 0)=w7394, index (dim 1)=w7393) -> (element=w7392:sgl[][][])  [unwired: 3 in]
                        n1822 = Equal?(x=w7391, y=w7408) -> (x = y?=w7407:bool)
                        n1823 = Equal?(x=w7389, y=w7408) -> (x = y?=w7405:bool)
                        n1824 = Equal?(x=w7390, y=w7408) -> (x = y?=w7403:bool)
                        n1825 = And(x=w7406, y=w7407) -> (x .and. y?=w7401:bool)
                        n1826 = And(x=w7404, y=w7405) -> (x .and. y?=w7400:bool)
                        n1827 = And(x=w7402, y=w7403) -> (x .and. y?=w7399:bool)
                        n1828 = Compound Arithmetic op=OR(w7401, w7400, w7399) -> (w7398:bool)
                        n1829 = case shown="True" w7398 {
                          tunnel: w7412 -> [w7418 w7422]
                          tunnel: w7411 -> [w7417 w7421]
                          tunnel: [w7415 w7420] -> w7410
                          tunnel: [w7416 w7419] -> w7409
                          tunnel: w7396 -> [w7414 _]
                          tunnel: w7392 -> [w7413 _]
                          frame False {
                            n1830 = Build Array (concatenate)(w7414, w7418) -> (w7415:sgl[])
                            n1831 = Build Array (concatenate)(w7413, w7417) -> (w7416:sgl[][][])
                            n1832 = local write "FI grid array"(w7416) -> ()
                            n1833 = local write "FI array"(w7415) -> ()
                          }
                          frame True {
                            n1834 = Build Array(w7422) -> (w7420:sgl[])
                            n1835 = Build Array(w7421) -> (w7419:sgl[][][])
                            n1836 = local write "FI array"(w7420) -> ()
                            n1837 = local write "FI grid array"(w7419) -> ()
                          }
                        }
                      }
                    }
                  }
                }
                n1838 = local write "FI array tiled"(w7363) -> ()
                n1839 = local write "FI grid array tiled"(w7362) -> ()
              }
              frame #23 {
                w7444 = 1000 ("sample length")
                n1840 = local read "SEM Options"() -> (w7449:T27)
                n1841 = Unbundle By Name(w7449) -> ("Upload"=w7448:bool)
                n1842 = local read "Smart upload fail"() -> (w7472:bool)
                n1843 = local read "Milling Z voltage array"() -> (w7443:sgl[])
                n1844 = local read "Milling Z voltage (V)"() -> (w7451:sgl)
                n1845 = Compound Arithmetic op=AND(w7448, "Smart upload", w7472) -> (w7473:bool)
                n1846 = Build Array (concatenate)(w7443, w7451) -> (w7470:sgl[])
                n1847 = case shown="True" w7473 {
                  frame False {
                  }
                  frame True {
                    n1848 = local read "SEM Scan Parameters"() -> (w7478:T26)
